vi "fileWrite.vi"() -> ()   [LabVIEW 2014]
panel:
  in  "Number of Values to Write":i32(knob)=20 scale=0.0..200.0
  out "File I/O Error":errorcluster
  in  "Browse For File":path
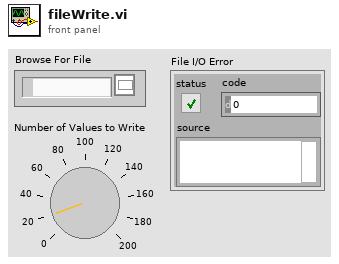
[diagram p1: front panel]
types:
  T1 = enum16{"open", "replace", "create", "open or create", "replace or create", "replace or create with confirmation"}
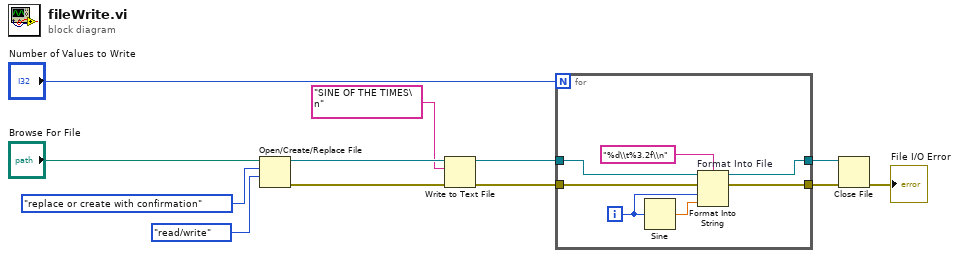
[diagram p0: block diagram]
diagram:
  n1 = Open/Create/Replace File(file path (use dialog)="Browse For File", operation (0:open)=T1."replace or create with confirmation", access (0:read/write)=enum16{"read/write", "read-only", "write-only"}."read/write") -> (refnum out=w11:refnum<file>, error out=w10:errorcluster)  [unwired: 3 in, 1 out]
  n2 = Write to Text File(file (use dialog)=w11, text="SINE OF THE TIMES\n", error in=w10) -> (refnum out=w3:refnum<file>, error out=w5:errorcluster)  [unwired: 1 in, 1 out]
  n3 = for {
    N: "Number of Values to Write" -> [_]
    tunnel: w5 -> [w17]
    tunnel: [w16] -> w4
    tunnel: w3 -> [w15]
    tunnel: [w14] -> w2
    i -> [w19]
    n4 = Sine(x=w19) -> (sin(x)=w18:dbl)
    n5 = Format Into String "Format Into File"(format string="%d\\t%3.2f\\n", initial string=w15, error in=w17, w19, w18) -> (resulting string=w14:refnum<file>, error out=w16:errorcluster)
  }
  n6 = Close File(refnum=w2, error in=w4) -> (error out=→"File I/O Error":errorcluster)  [unwired: 1 out]
